vi "read_data.vi"(8 "error in (no error)":errorcluster, 11 "GaussianProcessClassifier in":refnum<class "GaussianProcessClassifier.lvclass">) -> (0 "error out":errorcluster, 2 "data":T1={"y"=[], "sample_weight"=[], "clone_kernel"=TRUE}, 3 "GaussianProcessClassifier out":refnum<class "GaussianProcessClassifier.lvclass">)   [LabVIEW 2020, in "GaussianProcessClassifier.lvclass"]
uses:
  GaussianProcessClassifier.lvclass
  Controls/gaussian_process_classifier_data.ctl
  GaussianProcessClassifier.lvclass/GaussianProcessClassifier.ctl
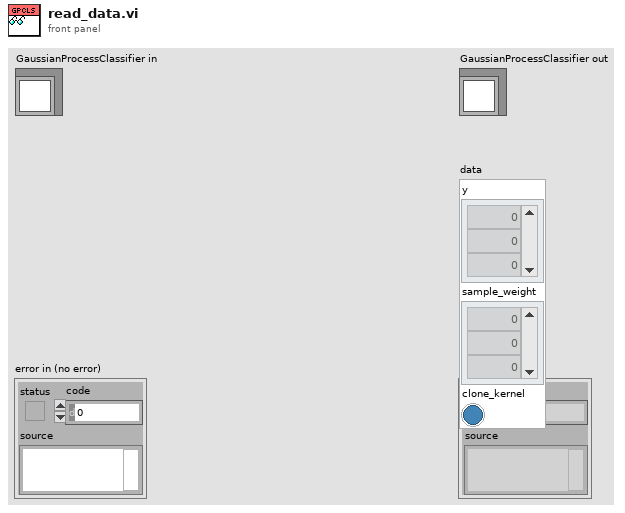
[diagram p1: front panel]
types:
  T1 = typedef "gaussian_process_classifier_data.ctl" = cluster{"y":dbl[], "sample_weight":dbl[], "clone_kernel":bool}
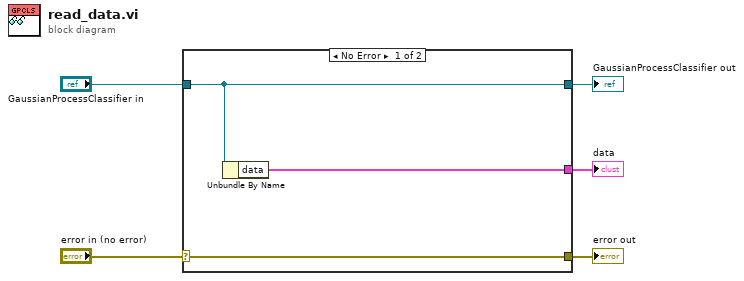
[diagram p0: block diagram]
diagram:
  n1 = case shown="No Error" "error in (no error)" {
    selector: "error in (no error)" -> [w8 w9]
    tunnel: [w8 w9] -> w4
    tunnel: [w7 w10] -> w2
    tunnel: "GaussianProcessClassifier in" -> [w7 w10]
    tunnel: [w6 _] -> w1
    frame No Error {
      n2 = Unbundle By Name(w7) -> ("data"=w6:T1)
    }
    frame Error {
    }
  }
  "error out" <- w4
  "GaussianProcessClassifier out" <- w2
  "data" <- w1
